vi "plot.volumes.vi"(4 "plot end":timestamp, 6 "plot start":timestamp, 7 "picture in":picture, 9 "Width":u32, 10 "rows":T1(array[cluster]), 11 "volume objects":cluster{"Array":T2[]}[](array[cluster])) -> (3 "picture":picture)   [LabVIEW 2024]
uses:
  volume.object--cluster.ctl
  definitions/volume.type--enum.ctl
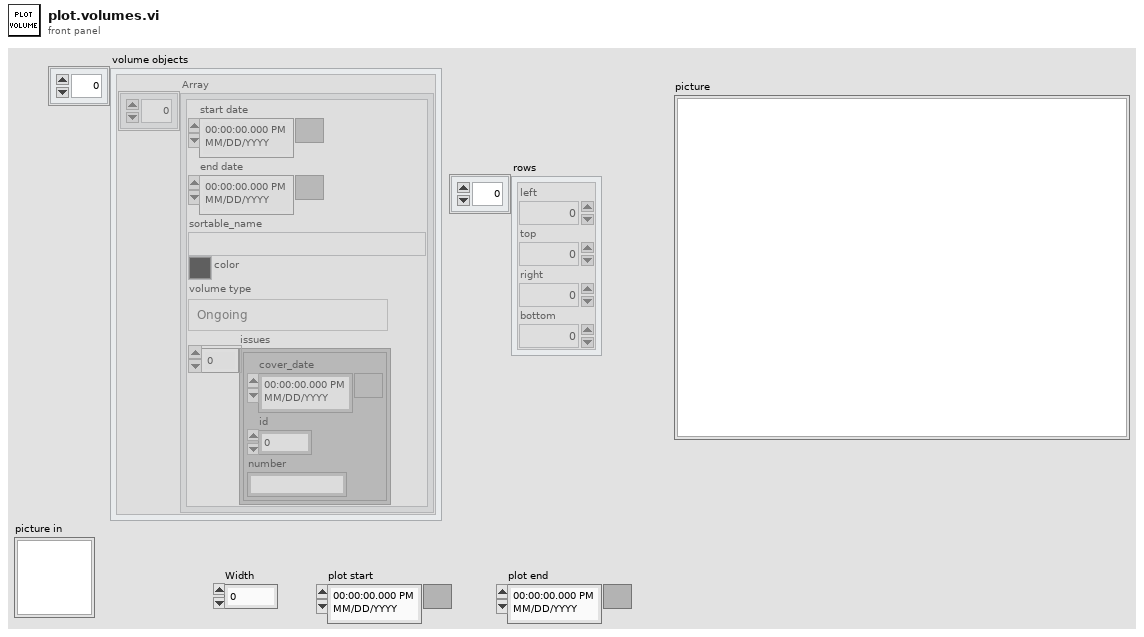
[diagram p1: front panel]
types:
  T1 = cluster{"left":i16, "top":i16, "right":i16, "bottom":i16}[]
  T2 = typedef "volume.object--cluster.ctl" = cluster{"start date":timestamp, "end date":timestamp, "sortable_name":string, "color":u32, "volume type":T3, "issues":cluster{"cover_date":timestamp, "id":i32, "number":string}[]}
  T3 = typedef "volume.type--enum.ctl" = enum16{"Ongoing", "Limited Series", "Annual", "One Shot", "Reprint/Document", "Star Comics", "Epic Comics"}
  T4 = cluster{"cover_date":timestamp, "id":i32, "number":string}[]
  T5 = cluster{"left":i16, "top":i16, "right":i16, "bottom":i16}
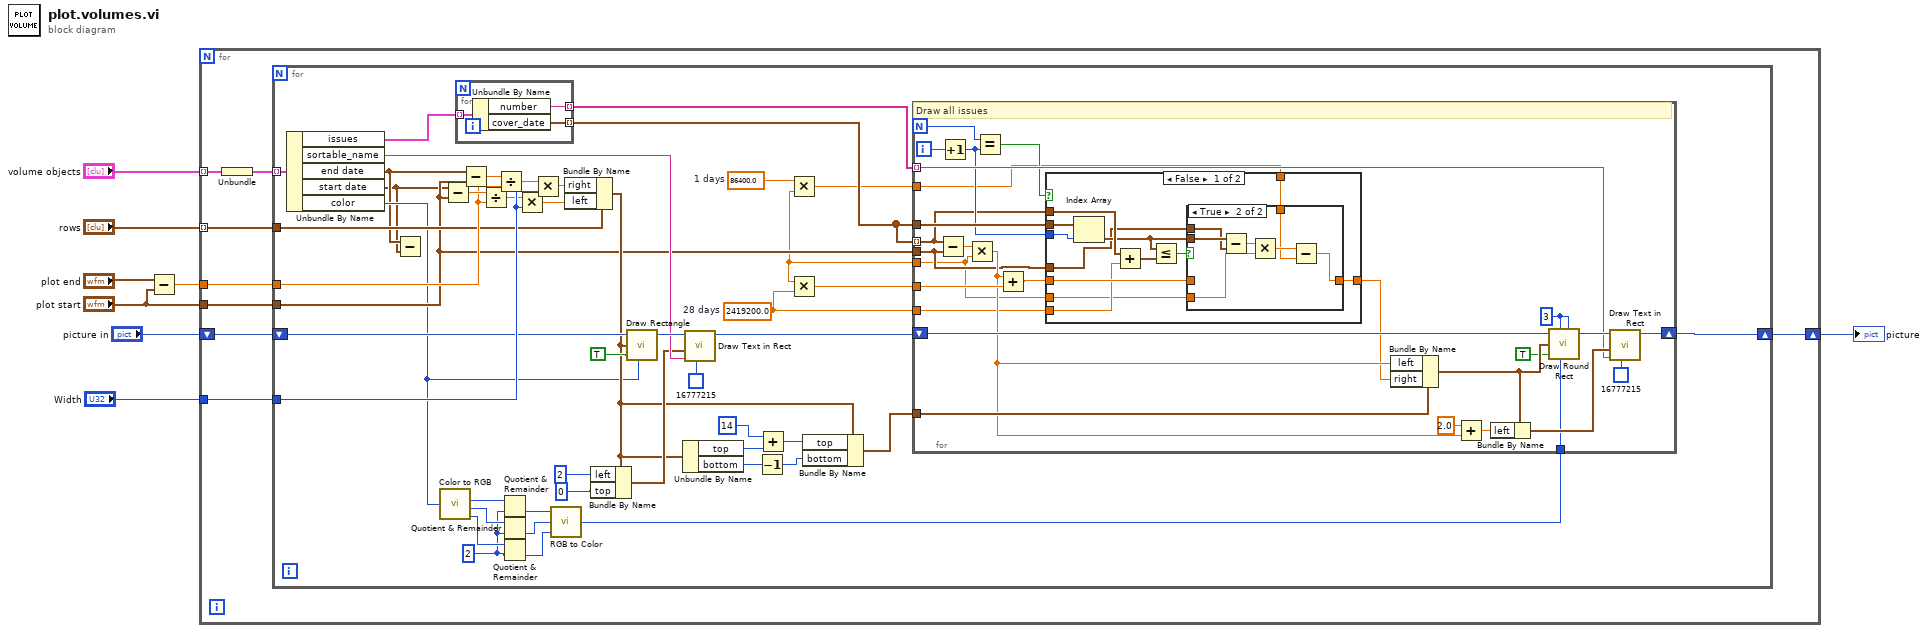
[diagram p0: block diagram]
diagram:
  n1 = Subtract(x="plot end", y="plot start") -> (x-y=w5:dbl)
  n2 = for {
    tunnel: "volume objects" -> [w16] mode=indexing
    tunnel: "rows" -> [w14] mode=indexing
    tunnel: w5 -> [w13]
    tunnel: "plot start" -> [w12]
    tunnel: "Width" -> [w11]
    shift-right: [w9] -> w2
    shift-left: "picture in" -> [w10]
    n3 = Unbundle(w16) -> ("Array"=w15:T2[])
    n4 = for {
      tunnel: w15 -> [w63] mode=indexing
      tunnel: w14 -> [w56]
      tunnel: w13 -> [w59]
      tunnel: w12 -> [w35]
      tunnel: w11 -> [w57]
      shift-right: [w20] -> w9
      shift-left: w10 -> [w53]
      w26 = u8 2 ("y")
      w30 = 2419200.0  # 28 days
      w34 = 86400.0  # 1 days
      n5 = Unbundle By Name(w63) -> ("issues"=w62:T4, "sortable_name"=w50:string, "end date"=w18:timestamp, "start date"=w17:timestamp, "color"=w22:u32)
      n6 = Subtract(x=w18, y=w17) -> ()  [unwired: 1 out]
      n7 = call <vilib>:"Color to RGB.vi"("Color"=w22) -> ("R"=w29:u8, "G"=w28:u8, "B"=w27:u8)  [unwired: 1 out]
      n8 = Subtract(x=w17, y=w35) -> (x-y=w60:dbl)
      n9 = for {
        tunnel: w62 -> [w115] mode=indexing
        tunnel: [w114] -> w44 mode=indexing
        tunnel: [w113] -> w36 mode=indexing
        n10 = Unbundle By Name(w115) -> ("number"=w114:string, "cover_date"=w113:timestamp)
      }
      n11 = Subtract(x=w18, y=w35) -> (x-y=w61:dbl)
      n12 = Divide(x=w60, y=w59) -> (x/y=w32:dbl)
      n13 = Divide(x=w61, y=w59) -> (x/y=w58:dbl)
      n14 = Quotient & Remainder(x=w29, y=w26) -> (floor(x/y)=w25:u8)  [unwired: 1 out]
      n15 = Quotient & Remainder(x=w28, y=w26) -> (floor(x/y)=w24:u8)  [unwired: 1 out]
      n16 = Quotient & Remainder(x=w27, y=w26) -> (floor(x/y)=w23:u8)  [unwired: 1 out]
      n17 = Multiply(x=w32, y=w57) -> (x*y=w55:dbl)
      n18 = Multiply(x=w58, y=w57) -> (x*y=w54:dbl)
      n19 = call <vilib>:"RGB to Color.vi"("B"=w23, "G"=w24, "R"=w25) -> ("Color"=w21:u32)
      n20 = Bundle By Name(cluster=w56, "right"=w54, "left"=w55) -> (w39:T5)
      n21 = Bundle By Name(cluster=w39, "left"=i16 2, "top"=i16 0) -> (w47:T5)
      n22 = call <vilib>:"Draw Rectangle.vi"("picture"=w53, "rect"=w39, "fill?(F)"=TRUE, "color(black)"=w22) -> ("new picture"=w51:picture)  [unwired: 5 in]
      n23 = Unbundle By Name(w39) -> ("top"=w43:i16, "bottom"=w41:i16)
      n24 = call <vilib>:"Draw Text in Rect.vi"("text color(black)"=u32 16777215, "text"=w50, "rect"=w47, "picture"=w51) -> ("new picture"=w45:picture)  [unwired: 7 in]
      n25 = Decrement(x=w41) -> (x-1=w38:i16)
      n26 = Add(x=i16 14, y=w43) -> (x+y=w40:i16)
      n27 = Multiply(x=w34) -> (y=w19:dbl, x*y=w33:dbl)
      n28 = Multiply(x=w19, y=w30) -> (x*y=w31:dbl)
      n29 = Bundle By Name(cluster=w39, "top"=w40, "bottom"=w38) -> (w37:T5)
      n30 = for {
        N -> [w74]
        tunnel: w19 -> [w65]
        tunnel: w35 -> [w66]
        tunnel: w31 -> [w90]
        tunnel: w37 -> [w89]
        shift-right: [w80] -> w20
        shift-left: w45 -> [w88]
        tunnel: w44 -> [w77] mode=indexing
        tunnel: w36 -> [w67] mode=indexing
        tunnel: w21 -> [w76]
        tunnel: w36 -> [w70]
        tunnel: w33 -> [w64]
        tunnel: w30 -> [w68]
        i -> [w75]
        w87 = i16 3 ("oval width")
        # "Draw all issues"
        n31 = Subtract(x=w67, y=w66) -> (x-y=w91:dbl)
        n32 = Increment(x=w75) -> (x+1=w69:i32)
        n33 = Multiply(x=w91, y=w65) -> (x*y=w86:dbl)
        n34 = Equal?(x=w74, y=w69) -> (x = y?=w73:bool)
        n35 = Add(x=w86, y=w90) -> (x+y=w71:dbl)
        n36 = case shown="False" w73 {
          tunnel: [w100 w112] -> w72
          tunnel: w71 -> [w99 w112]
          tunnel: w70 -> [w103 _]
          tunnel: w69 -> [w102 _]
          tunnel: w68 -> [w98 _]
          tunnel: w67 -> [w96 _]
          tunnel: w66 -> [w94 _]
          tunnel: w65 -> [w93 _]
          tunnel: w64 -> [w92 _]
          frame False {
            n37 = Index Array(array=w103, index=w102) -> (element=w95:timestamp)
            n38 = Add(x=w96, y=w98) -> (x+y=w97:timestamp)
            n39 = Less Or Equal?(x=w95, y=w97) -> (x <= y?=w101:bool)
            n40 = case shown="True" w101 {
              tunnel: [w104 w105] -> w100
              tunnel: w99 -> [w104 _]
              tunnel: w95 -> [_ w111]
              tunnel: w94 -> [_ w110]
              tunnel: w93 -> [_ w108]
              tunnel: w92 -> [_ w106]
              frame False {
              }
              frame True {
                n41 = Subtract(x=w111, y=w110) -> (x-y=w109:dbl)
                n42 = Multiply(x=w109, y=w108) -> (x*y=w107:dbl)
                n43 = Subtract(x=w107, y=w106) -> (x-y=w105:dbl)
              }
            }
          }
          frame True {
          }
        }
        n44 = Bundle By Name(cluster=w89, "left"=w86, "right"=w72) -> (w83:T5)
        n45 = Add(x=2.0, y=w86) -> (x+y=w84:dbl)
        n46 = Bundle By Name(cluster=w83, "left"=w84) -> (w79:T5)
        n47 = call <vilib>:"Draw Round Rect.vi"("picture"=w88, "oval width"=w87, "rect"=w83, "fill?(F)"=TRUE, "color(black)"=w76, "oval height"=w87) -> ("new picture"=w81:picture)  [unwired: 3 in]
        n48 = call <vilib>:"Draw Text in Rect.vi"("text color(black)"=u32 16777215, "text"=w77, "rect"=w79, "picture"=w81) -> ("new picture"=w80:picture)  [unwired: 7 in]
      }
    }
  }
  "picture" <- w2
